vi "get_current_range_offset_values.vi"(8 "error in (no error)":errorcluster, 11 "DL090216RangeOffsetImageProcessor in":refnum<class "ImageProcessorDL090216RangeOffset.lvclass">) -> (0 "error out":errorcluster, 2 "range offset values (channels)":T1[](array[typedef]) {"offset" min=0.0 max=1.0 step=0.0010000000474974513 scale=0.0..1.0; "range" min=0.0 max=1.0 step=0.0010000000474974513 scale=0.0..1.0}, 3 "DL090216RangeOffsetImageProcessor out":refnum<class "ImageProcessorDL090216RangeOffset.lvclass">)   [LabVIEW 2010, in "ImageProcessorDL090216RangeOffset.lvclass"]
uses:
  ImageProcessorDL090216RangeOffset.lvclass
  common/clusters/range_offset_cluster.ctl
  ImageProcessorDL090216RangeOffset.lvclass/ImageProcessorDL090216RangeOffset.ctl
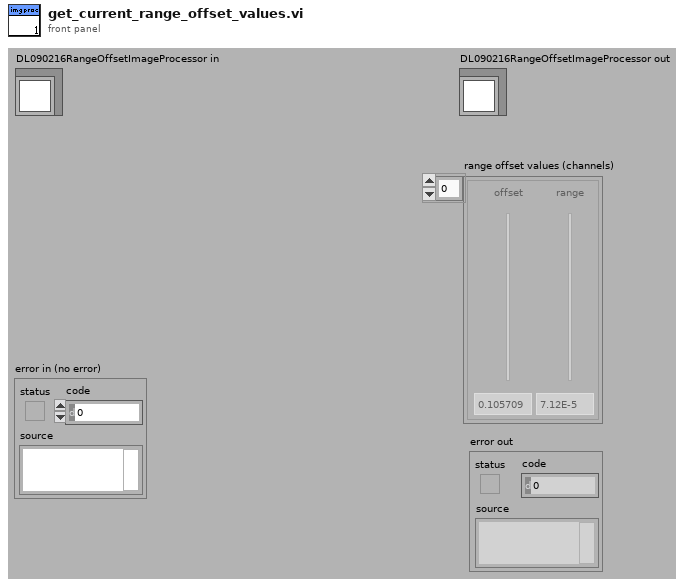
[diagram p1: front panel]
types:
  T1 = typedef "range_offset_cluster.ctl" = cluster{"range":dbl, "offset":dbl}
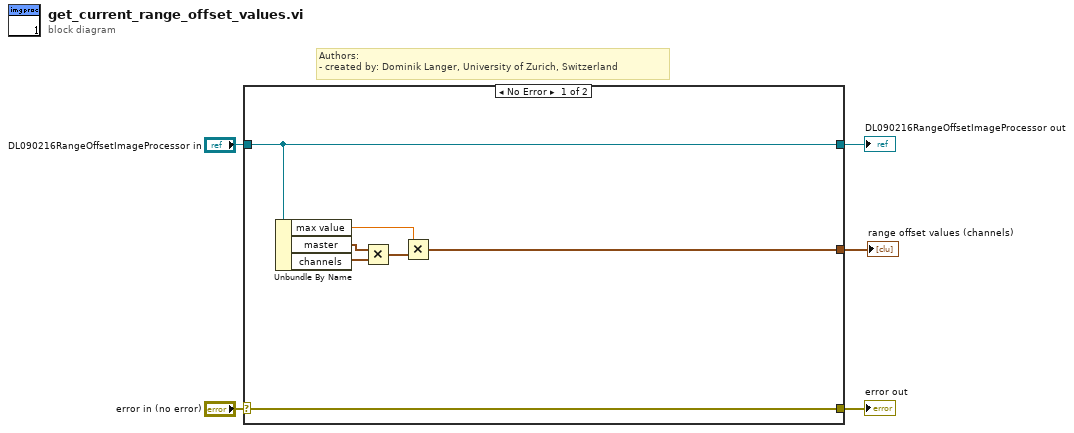
[diagram p0: block diagram]
diagram:
  # "Authors: \n- created by: Dominik Langer, University of Zurich, Switzerland"
  n1 = case shown="No Error" "error in (no error)" {
    selector: "error in (no error)" -> [w12 w14]
    tunnel: [w12 w14] -> w4
    tunnel: [w7 w13] -> w2
    tunnel: "DL090216RangeOffsetImageProcessor in" -> [w7 w13]
    tunnel: [w6 _] -> w1
    frame No Error {
      n2 = Unbundle By Name(w7) -> ("max value"=w8:dbl, "master"=w10:T1, "channels"=w11:T1[])
      n3 = Multiply(x=w10, y=w11) -> (x*y=w9:T1[])
      n4 = Multiply(x=w8, y=w9) -> (x*y=w6:T1[])
    }
    frame Error {
    }
  }
  "error out" <- w4
  "DL090216RangeOffsetImageProcessor out" <- w2
  "range offset values (channels)" <- w1
